vi "LED_LUT.vi"(7 "reset":bool, 8 "Previous value of randomly generated testpulse separation":u32, 10 "seed":u32=4294967295, 11 "Need a new random number?":bool) -> (0 "Randomly generated testpulse separation out":u32)   [LabVIEW 2012]
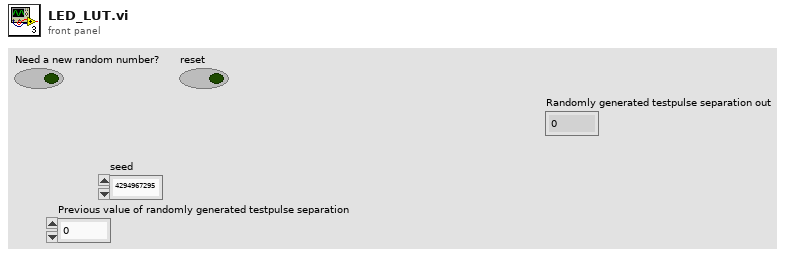
[diagram p1: front panel]
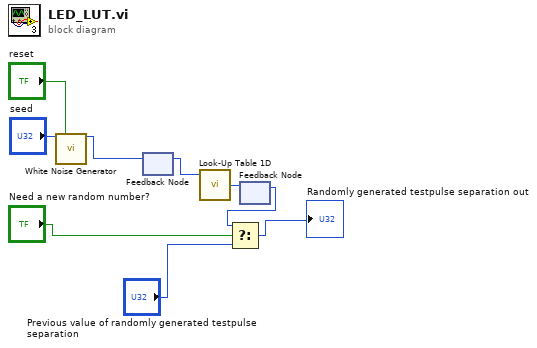
[diagram p0: block diagram]
diagram:
  n1 = call "White Noise Generator"("seed"="seed", "reset"="reset") -> ("white noise out"=w4:i16)  [unwired: 13 in]
  n2 = feedback-in #1(w4) -> ()
  n3 = feedback #1() -> (w3:i16)  [unwired: 1 in]
  n4 = call "Look-Up Table 1D"("address"=w3) -> ("data out"=w2:u32)  [unwired: 8 in]
  n5 = feedback #2() -> (w1:u32)  [unwired: 1 in]
  n6 = Select(t=w1, s="Need a new random number?", f="Previous value of randomly generated testpulse separation") -> (s? t:f=→"Randomly generated testpulse separation out":u32)
  n7 = feedback-in #2(w2) -> ()
